vi "Read File Path.vi"(8 "error in (no error)":errorcluster, 11 "File Path Result in":refnum<class "File Path Result.lvclass">) -> (0 "error out":errorcluster, 2 "File Path":path, 3 "File Path Result out":refnum<class "File Path Result.lvclass">)   [LabVIEW 2015, in "File Path Result.lvclass"]
uses:
  File Path Result.lvclass
  File Path Result.lvclass/File Path Result.ctl
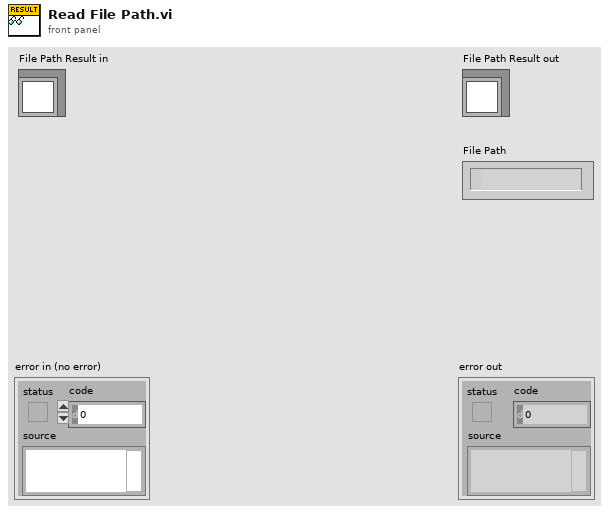
[diagram p1: front panel]
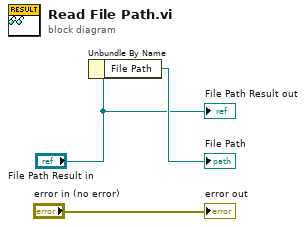
[diagram p0: block diagram]
diagram:
  n1 = Unbundle By Name("File Path Result in") -> ("File Path"=→"File Path":path)
  "error out" <- "error in (no error)"
  "File Path Result out" <- "File Path Result in"
